vi "GetWindowsDirectory.vi"() -> ()   [LabVIEW 2011]
doc: "Uses an API call to retrieve the path to the Windows directorye."
uses:
  kernel32.dll
panel:
  out "error out":errorcluster
  in  "error in (no error)":errorcluster
  out "Windows Path":string
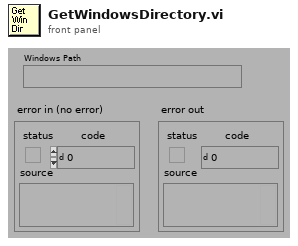
[diagram p1: front panel]
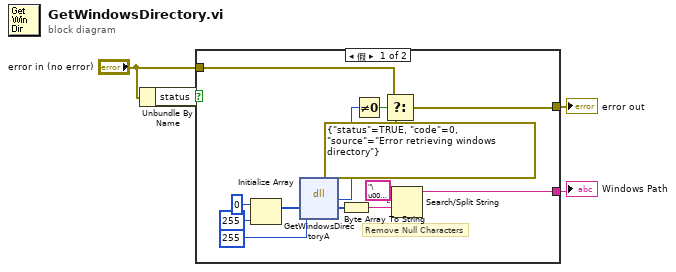
[diagram p0: block diagram]
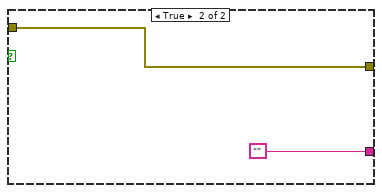
[diagram p2: hidden frame]
diagram:
  n1 = Unbundle By Name("error in (no error)") -> ("status"=w3:bool)
  n2 = case shown="假" w3 {
    tunnel: [w14 "" ("string")] -> w4
    tunnel: "error in (no error)" -> [w10 w19]
    tunnel: [w9 w19] -> w1
    frame False {
      # "Remove Null Characters"
      n3 = Initialize Array(u8 0, 255) -> (w7:u8[])
      n4 = dll-call lib="kernel32.dll" fn="GetWindowsDirectoryA" label="Get Windows Directory"("lpBuffer"=w7, "uSize"=u32 255 ("nSize")) -> (w12:u8, "lpBuffer"=w5:u8[])  [unwired: 4 in, 2 out]
      n5 = Byte Array To String(unsigned byte array=w5) -> (string=w16:string)
      n6 = Not Equal To 0?(x=w12) -> (x != 0?=w11:bool)
      n7 = Select(t=w10, s=w11, f=errorcluster {"status"=TRUE, "code"=0, "source"="Error retrieving windows directory"}) -> (s? t:f=w9:errorcluster)
      n8 = Search/Split String(string=w16, search string/char (-)="\u0000" ("regular expression")) -> (substring before match=w14:string)  [unwired: 1 in, 2 out]
    }
    frame True {
    }
  }
  "Windows Path" <- w4
  "error out" <- w1
